vi "Lab4.vi"() -> ()   [LabVIEW 2011]
panel:
  in  "stop":bool
  out "?":dbl
  out "vlaoarea Instantanee":dbl(graph)
  in  "diametru":dbl(slide)=4.0 scale=0.0..10.0
  out "Volum":dbl(slide) scale=0.0..550.0
  out "Variatia Inaltimii":dbl(knob) scale=0.0..11.0
  out "?":dbl=5.0
  in  "Inaltime":dbl(slide)=4.451612903225806 scale=0.0..10.0 scale format="%#.2g"
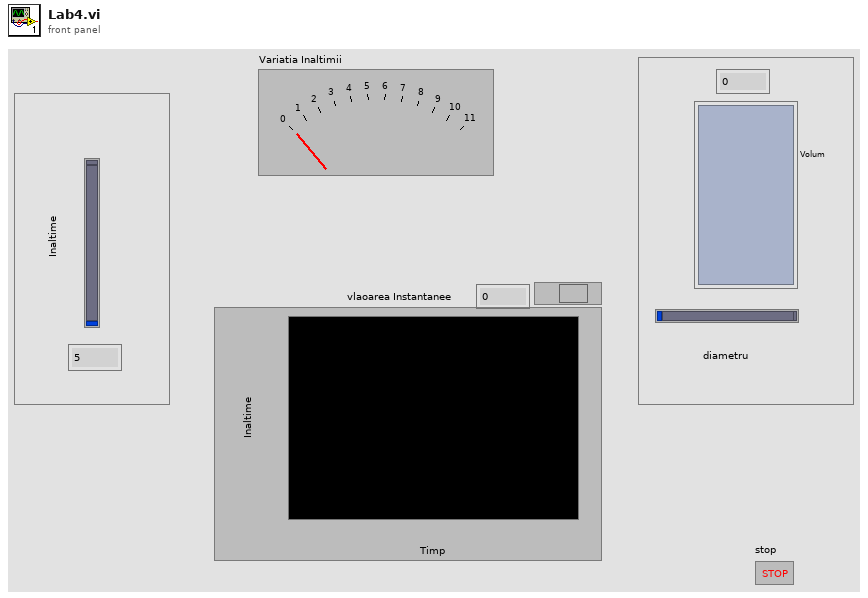
[diagram p1: front panel]
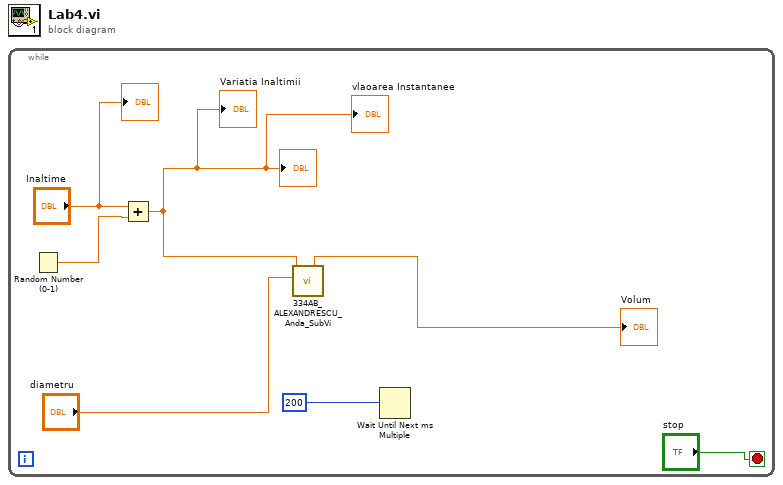
[diagram p0: block diagram]
diagram:
  n1 = while {
    stop <- "stop" stop-if-true
    n2 = Random Number (0-1)() -> (number: 0 to 1=w4:dbl)
    n3 = Add(x="Inaltime", y=w4) -> (x+y=w2:dbl)
    "Variatia Inaltimii" <- w2
    "vlaoarea Instantanee" <- w2
    "?" <- w2
    n4 = call "334AB_ALEXANDRESCU_Anda_SubVi.vi"("Diametru"="diametru", "Inaltime"=w2) -> ("Numeric"=→"Volum":dbl)  [unwired: 9 in]
    n5 = Wait Until Next ms Multiple(millisecond multiple=200) -> ()  [unwired: 1 out]
    "?" <- "Inaltime"
  }
